vi "send visualization command.vi"(8 "error in (no error)":errorcluster, 9 "data":variant, 10 "state":T1, 11 "Queue in":refnum<queue>) -> (0 "error out":errorcluster)   [LabVIEW 2016, in "FPGA Addon System Explorer.lvlib"]
uses:
  viz_state.ctl
  viz_command.ctl
  FPGA Addon System Explorer.lvlib
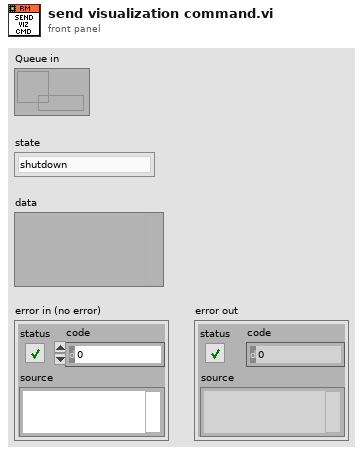
[diagram p1: front panel]
types:
  T1 = typedef "FPGA Addon System Explorer.lvlib/viz_state.ctl" = enum16{"shutdown"}
  T2 = typedef "FPGA Addon System Explorer.lvlib/viz_command.ctl" = cluster{"state":T1, "data":variant}
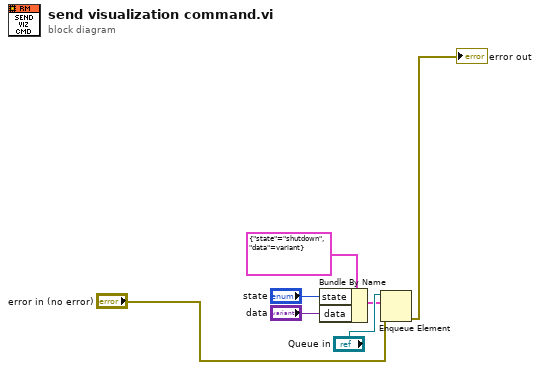
[diagram p0: block diagram]
diagram:
  n1 = Bundle By Name(cluster=T2 {"state"=enum."shutdown", "data"=variant} ("viz_command"), "state"="state", "data"="data") -> (w3:T2)
  n2 = Enqueue Element(queue="Queue in", element=w3, error in (no error)="error in (no error)") -> (error out=→"error out":errorcluster)  [unwired: 1 in, 2 out]
